vi "Add Header.vi"(8 "error in":errorcluster, 9 "value":string, 10 "header":string, 11 "REST Client in":refnum<class "REST Client.lvclass">) -> (0 "error out":errorcluster, 3 "REST Client out":refnum<class "REST Client.lvclass">)   [LabVIEW 2020, in "REST Client.lvlib" / "REST Client.lvclass"]
uses:
  REST Client.lvclass
  REST Client.lvclass/REST Client.ctl
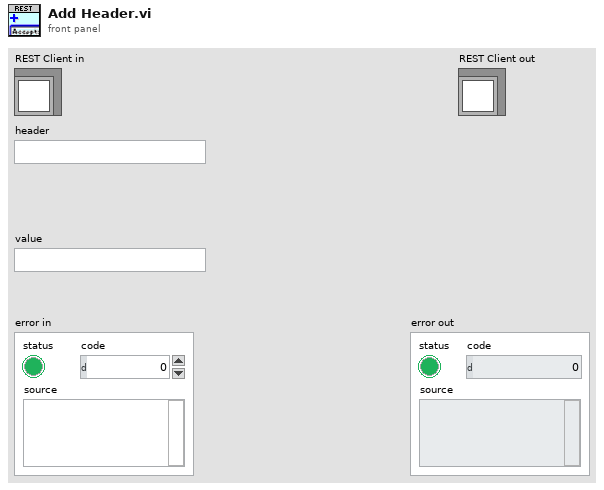
[diagram p1: front panel]
types:
  T1 = typedef "REST Client.lvlib/REST Client.lvclass/HTTP Header.ctl" = cluster{"header":string, "value":string}
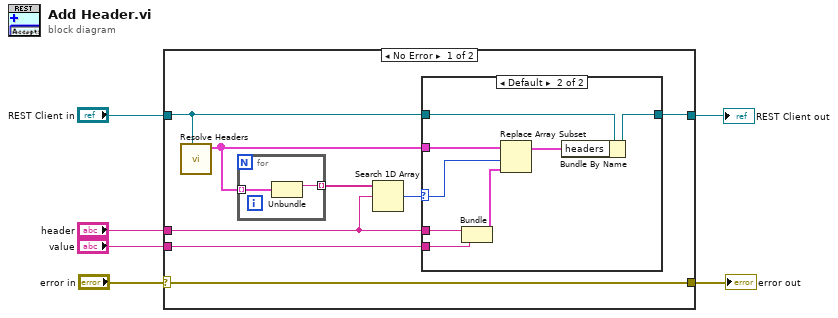
[diagram p0: block diagram]
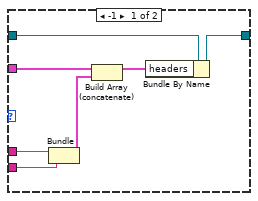
[diagram p2: hidden frame]
diagram:
  n1 = case shown="No Error" "error in" {
    selector: "error in" -> [w10 w32]
    tunnel: "header" -> [w7 _]
    tunnel: "REST Client in" -> [w11 w33]
    tunnel: [w9 w33] -> w5
    tunnel: [w10 w32] -> w4
    tunnel: "value" -> [w8 _]
    frame No Error {
      n2 = call "Resolve Headers.vi"("REST Client in"=w11) -> ("headers out"=w12:T1[])  [unwired: 10 in]
      n3 = for {
        tunnel: w12 -> [w31] mode=indexing
        tunnel: [w30] -> w13 mode=indexing
        n4 = Unbundle(w31) -> ("header"=w30:string)  [unwired: 1 out]
      }
      n5 = Search 1D Array(1D array=w13, element=w7) -> (index of element=w14:i32)  [unwired: 1 in]
      n6 = case shown="Default" w14 {
        selector: w14 -> [_ w24]
        tunnel: w12 -> [w19 w25]
        tunnel: w11 -> [w20 w28]
        tunnel: [w21 w29] -> w9
        tunnel: w8 -> [w18 w27]
        tunnel: w7 -> [w17 w26]
        frame -1 {
          n7 = Bundle("header"=w17, "value"=w18) -> (w16:cluster{"header":string, "value":string})  [unwired: 1 in]
          n8 = Build Array (concatenate)(w19, w16) -> (w15:T1[])
          n9 = Bundle By Name(cluster=w20, "headers"=w15) -> (w21:refnum<class "REST Client.lvclass">)
        }
        frame Default {
          n10 = Bundle("header"=w26, "value"=w27) -> (w23:cluster{"header":string, "value":string})  [unwired: 1 in]
          n11 = Replace Array Subset(array=w25, new element=w23, index=w24) -> (w22:T1[])
          n12 = Bundle By Name(cluster=w28, "headers"=w22) -> (w29:refnum<class "REST Client.lvclass">)
        }
      }
    }
    frame Error {
    }
  }
  "error out" <- w4
  "REST Client out" <- w5
